vi "TM_lab2.vi"() -> ()   [LabVIEW 2014]
uses:
  <vilib>/Utility/file.llb/Write To Spreadsheet File (DBL).vi
panel:
  in  "Analog Input Commands":T1={"Channels"=[0, 0, 0, 0], "Gains (Diff Only)"=[0, 0, 0, 0], "Number of Channels (1,2,4)"=1} {"Gains (Diff Only)" items=["1 (+/-20V)", "2 (+/-10V)", "4 (+/-5V)", "5 (+/-4V)", "8 (+/-2.5V)", "10 (+/-2V)", "16 (+/-1.25V)", "20 (+/-1V)"]; "Channels" items=["0 SE (+/-10V)", "1 SE (+/-10V)", "2 SE (+/-10V)", "3 SE (+/-10V)", "4 SE (+/-10V)", "5 SE (+/-10V)", "6 SE (+/-10V)", "7 SE (+/-10V)", "0-1 Diff", "2-3 Diff", "4-5 Diff", "6-7 Diff"]}
  in  "error in":errorcluster
  in  "IDNum (-1)":i32=-1
  out "Local ID":i32
  in  "file path (dialog if empty)":path
  out "Array":dbl[][](array[numeric])
  out "Error":string
  out "Analog Input Data":T2 {"Voltages" format="%.4f"}
  in  "stop":bool
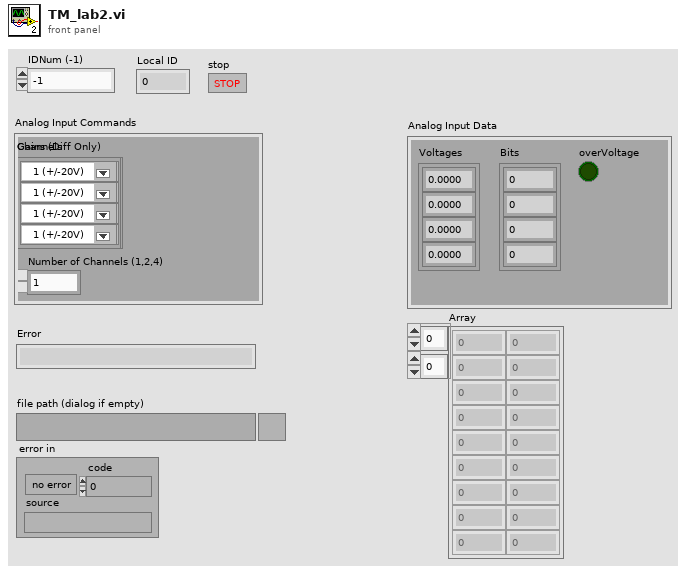
[diagram p1: front panel]
types:
  T1 = cluster{"Channels":u16[], "Gains (Diff Only)":u16[], "Number of Channels (1,2,4)":i32}
  T2 = cluster{"Voltages":dbl[], "Bits":i32[], "overVoltage":bool}
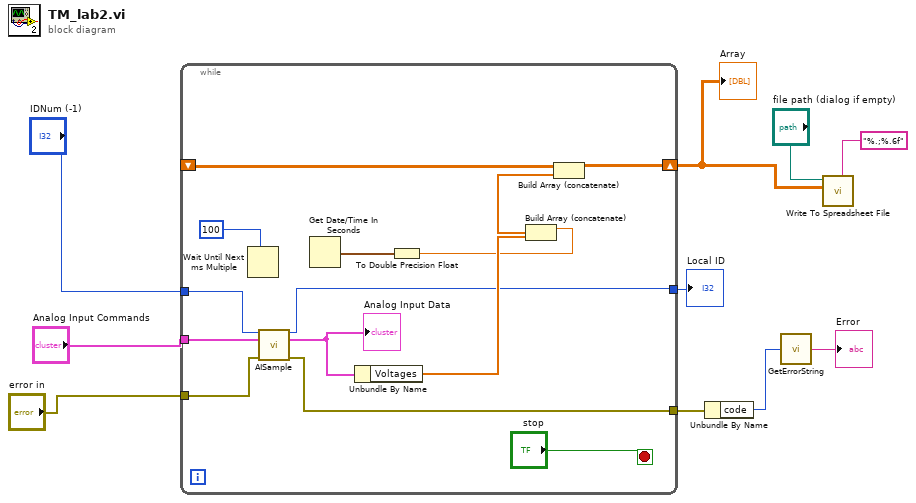
[diagram p0: block diagram]
diagram:
  n1 = while {
    tunnel: "IDNum (-1)" -> [w24]
    tunnel: "error in" -> [w23]
    tunnel: "Analog Input Commands" -> [w22]
    tunnel: [w21] -> w8
    shift-right: [w14] -> w7
    shift-left: _ -> [w12]
    tunnel: [w11] -> w5
    stop <- "stop" stop-if-true
    n2 = Wait Until Next ms Multiple(millisecond multiple=u32 100) -> ()  [unwired: 1 out]
    n3 = call "AISample.vi"("IDNum (-1)"=w24, "Analog Input Commands"=w22, "error in"=w23) -> ("Local ID"=w11:i32, "Analog Input Data"=w17:T2, "error out"=w21:errorcluster)  [unwired: 9 in, 1 out]
    "Analog Input Data" <- w17
    n4 = Get Date/Time In Seconds() -> (seconds since 1Jan1904=w18:timestamp)
    n5 = Unbundle By Name(w17) -> ("Voltages"=w16:dbl[])
    n6 = To Double Precision Float(number=w18) -> (double precision float=w15:dbl)
    n7 = Build Array (concatenate)(w15, w16) -> (w13:dbl[])
    n8 = Build Array (concatenate)(w12, w13) -> (w14:dbl[][])
  }
  "Array" <- w7
  "Local ID" <- w5
  n9 = Unbundle By Name(w8) -> ("code"=w10:i32)
  n10 = call "GetErrorString.vi"("Errorcode"=w10) -> ("Error"=→"Error":string)
  n11 = call-poly <vilib>:"Write To Spreadsheet File.vi"("format (%.3f)"="%.;%.6f", "2D data"=w7, "file path (dialog if empty)"="file path (dialog if empty)") -> ()  [unwired: 5 in, 1 out]
